vi "CRYChange Curve Library.vi"(4 "Waveform":T1={"Waveform"={"X0"=0.0, "dX"=0.0, "Y"=[]}, "X data"=1, "Y data"=1, "Y axis"=1, "X unit"="s", "Y unit"="V", "Y dB ref"=1.0, "display Y"=TRUE, "display X"=TRUE, "Overload?"=FALSE, "Test Info"="", "Step No."=0, "Name"="", "protected"=FALSE, "Sqc history"=[], "Signal Channel ID"=0, "Plot Settings"={"Color"=0, "Interpolation"=0, "Point Style"=0, "Line Style"=0, "Point Color"=0, "Line Width"=0, "Bar Plot Style"=0, "Fill To"=0}, "AutoProtect"=FALSE} {"Y dB ref" format="%.1f"; "Y axis" items=["Log", "Lin"]; "Y data" items=["dB", "Lin"]; "X data" items=["dB", "Lin"]}, 5 "sOptioin 2":string, 6 "Result":T2={"Name"="Test for Signal [L]", "Margin"=nan, "unit"="", "Verdict"=FALSE, "Limit"="", "Max/Min"="", "protected"=FALSE, "Step No."=0, "Test Info"="", "AutoProtect"=FALSE} {"Margin" format="%.2f"}, 7 "sOptioin 1":string, 8 "Index":i32[](array[numeric]), 9 "Curve":T3={"Name"="", "Curve"=[], "X data"=1, "Y data"=1, "Z data"=1, "X axis"=0, "Y axis"=1, "Z axis"=1, "X unit"="Hz", "Y unit"="", "Z unit"="deg.", "X dB ref"=1.0, "Y dB ref"=1.0, "Z dB ref"=1.0, "single val"=FALSE, "protected"=FALSE, "display X"=TRUE, "display Y"=TRUE, "display Z"=TRUE, "Test Info"="", "Step No."=0, "Plot Settings"={"Color"=0, "Interpolation"=0, "Point Style"=0, "Line Style"=0, "Point Color"=0, "Line Width"=0, "Bar Plot Style"=0, "Fill To"=0}, "AutoProtect"=FALSE} {"Z data" items=["dB", "Lin"]; "X data" items=["dB", "Lin"]; "Y data" items=["dB", "Lin"]; "Z dB ref" format="%.1f"; "Z axis" items=["Log", "Lin"]; "X dB ref" format="%.1f"; "X axis" items=["Log", "Lin"]; "Y axis" items=["Log", "Lin"]; "Y dB ref" format="%.1f"; "Curve"."z" format="%.2f"; "Curve"."y" format="%.2f"; "Curve"."x" format="%.2f"}, 10 "Type In":enum16{"Curves", "Values", "Results", "WFM"}(ring), 11 "sAction":string) -> (2 "Inserted index":i32[](array[numeric]), 3 "Name Out":string[](array[string]))   [LabVIEW 2013]
uses:
  CRYSystem/Typedef Control/CRYData Cluster.ctl
  CRYSystem/Typedef Control/CRYResult Cluster.ctl
  CRYSystem/Typedef Control/CRYWaveform Cluster.ctl
  CRYSystem/Task Sequence/CRYProject Run Control Global.vi
  Global/CRYCurve Library Global.vi
  Global/CRYCurves Array Global.vi
panel:
  # "Save All Data(Curves, Values,Results, Waveforms)"
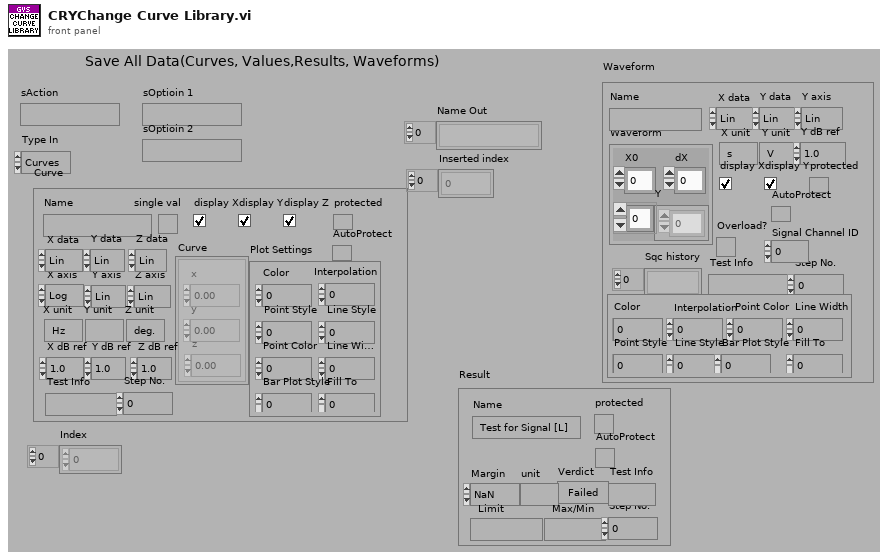
[diagram p1: front panel]
types:
  T1 = typedef "CRYWaveform Cluster.ctl" = cluster{"Waveform":cluster{"X0":dbl, "dX":dbl, "Y":sgl[]}, "X data":u16, "Y data":u16, "Y axis":u16, "X unit":string, "Y unit":string, "Y dB ref":dbl, "display Y":bool, "display X":bool, "Overload?":bool, "Test Info":string, "Step No.":i32, "Name":string, "protected":bool, "Sqc history":string[], "Signal Channel ID":i32, "Plot Settings":cluster{"Color":u32, "Interpolation":u8, "Point Style":u8, "Line Style":u8, "Point Color":u32, "Line Width":u8, "Bar Plot Style":u8, "Fill To":i16}, "AutoProtect":bool}
  T2 = typedef "CRYResult Cluster.ctl" = cluster{"Name":string, "Margin":dbl, "unit":string, "Verdict":bool, "Limit":string, "Max/Min":string, "protected":bool, "Step No.":i32, "Test Info":string, "AutoProtect":bool}
  T3 = typedef "CRYData Cluster.ctl" = cluster{"Name":string, "Curve":cluster{"x":dbl, "y":dbl, "z":dbl}[], "X data":u16, "Y data":u16, "Z data":u16, "X axis":u16, "Y axis":u16, "Z axis":u16, "X unit":string, "Y unit":string, "Z unit":string, "X dB ref":dbl, "Y dB ref":dbl, "Z dB ref":dbl, "single val":bool, "protected":bool, "display X":bool, "display Y":bool, "display Z":bool, "Test Info":string, "Step No.":i32, "Plot Settings":cluster{"Color":u32, "Interpolation":u8, "Point Style":u8, "Line Style":u8, "Point Color":u32, "Line Width":u8, "Bar Plot Style":u8, "Fill To":i16}, "AutoProtect":bool}
  T4 = typedef "CRYWaveform Cluster Array.ctl" = T1[]
  T5 = typedef "CRYResult Cluster Array.ctl" = T2[]
  T6 = typedef "CRYData Cluster Array.ctl" = T3[]
  T7 = cluster{"Color":u32, "Interpolation":u8, "Point Style":u8, "Line Style":u8, "Point Color":u32, "Line Width":u8, "Bar Plot Style":u8, "Fill To":i16}
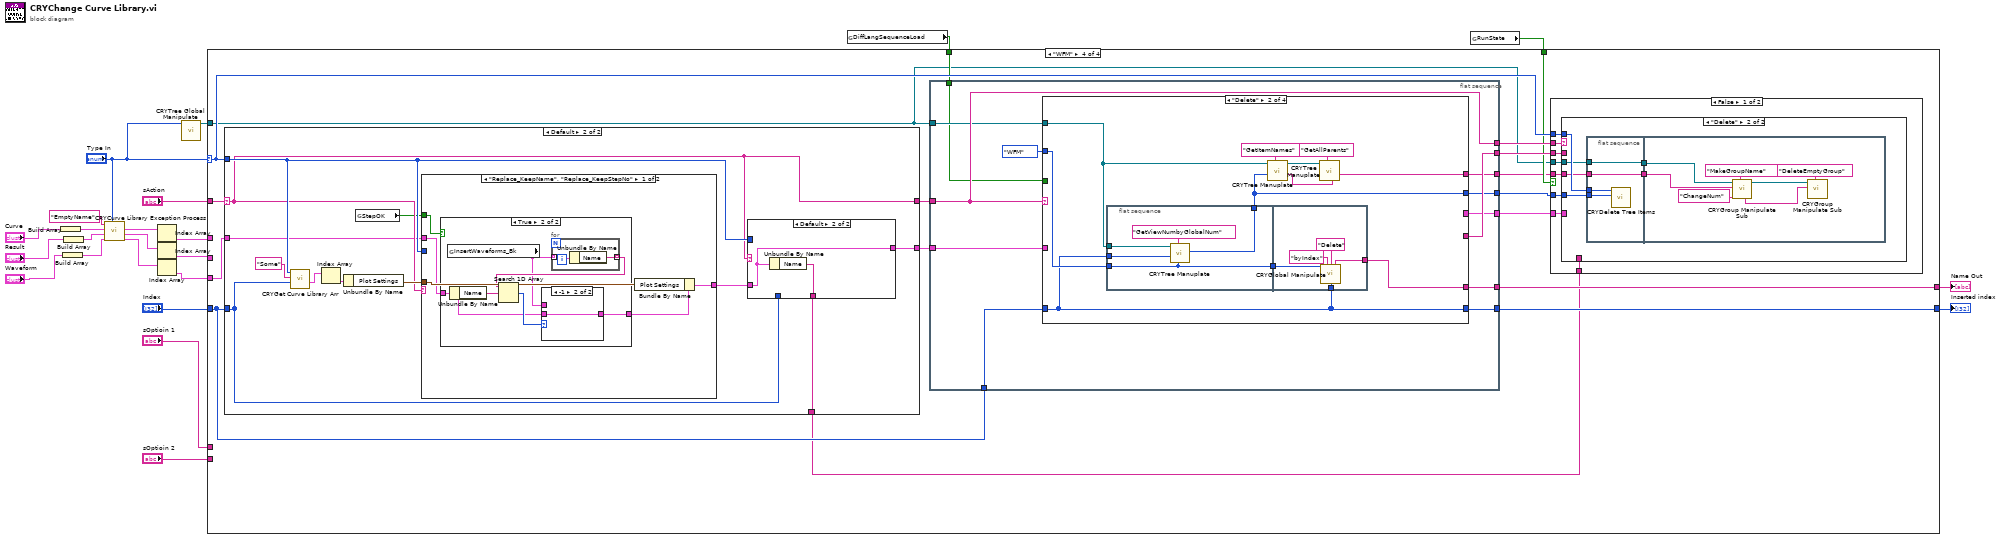
[diagram p0: block diagram]
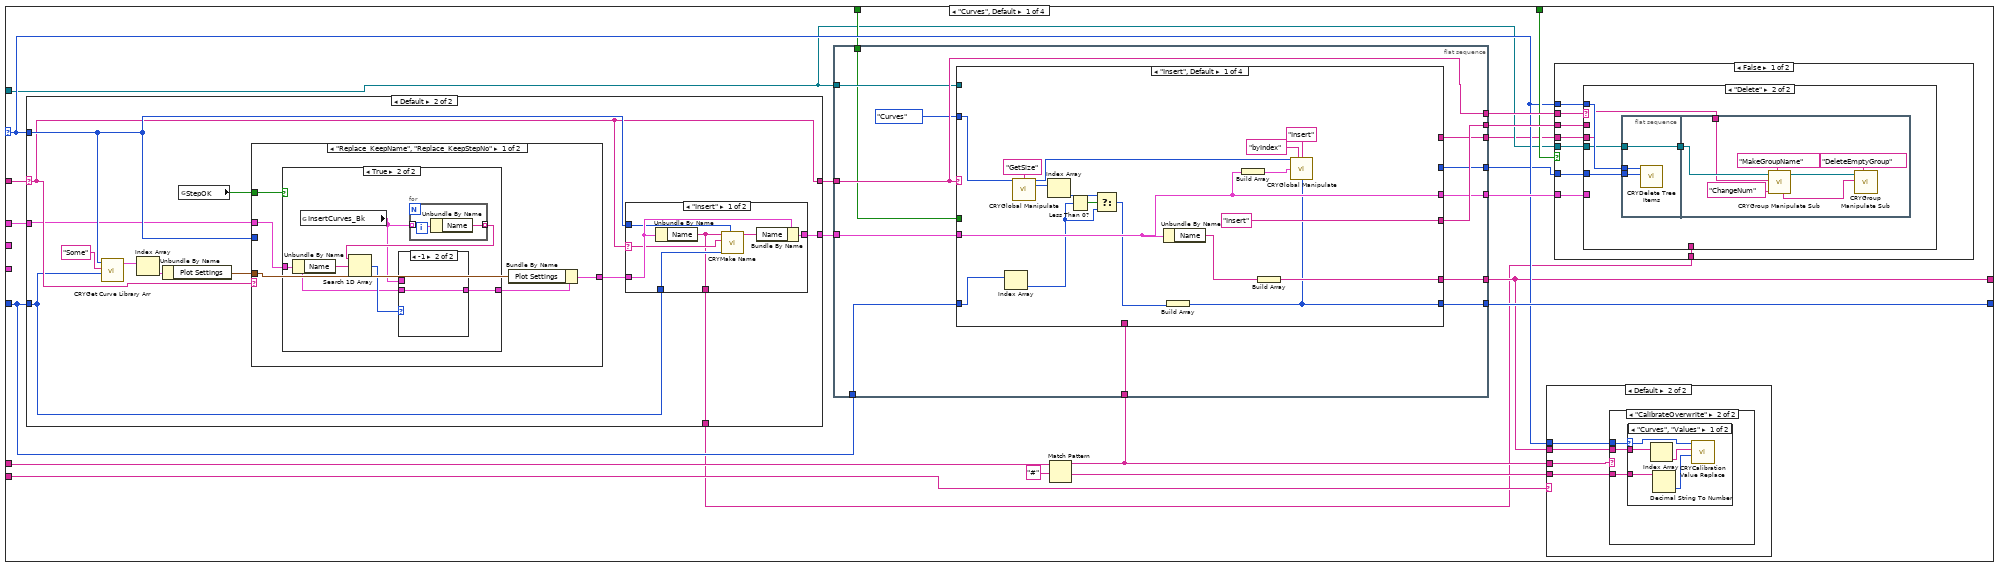
[diagram p2: hidden frame]
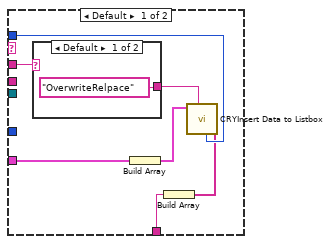
[diagram p6: hidden frame]
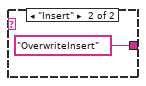
[diagram p7: hidden frame]
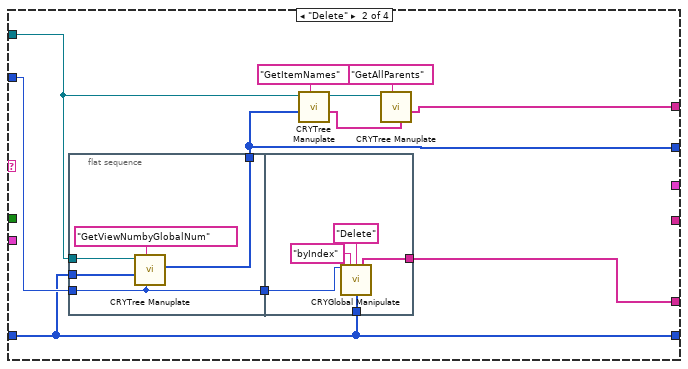
[diagram p9: hidden frame]
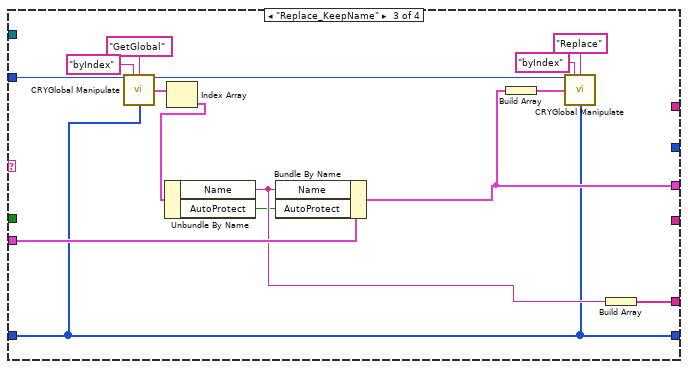
[diagram p10: hidden frame]
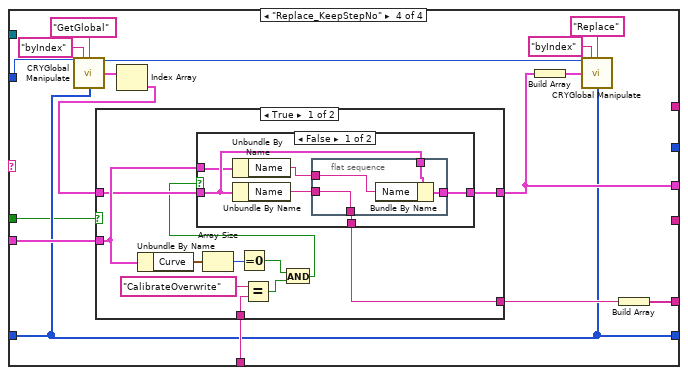
[diagram p11: hidden frame]
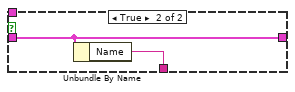
[diagram p12: hidden frame]
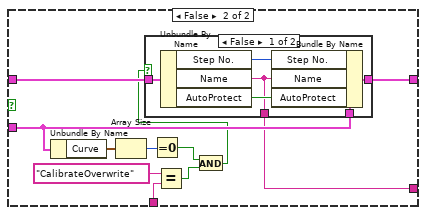
[diagram p13: hidden frame]
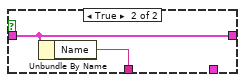
[diagram p14: hidden frame]
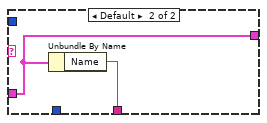
[diagram p16: hidden frame]
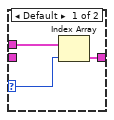
[diagram p18: hidden frame]
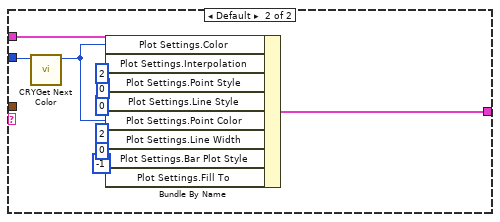
[diagram p19: hidden frame]
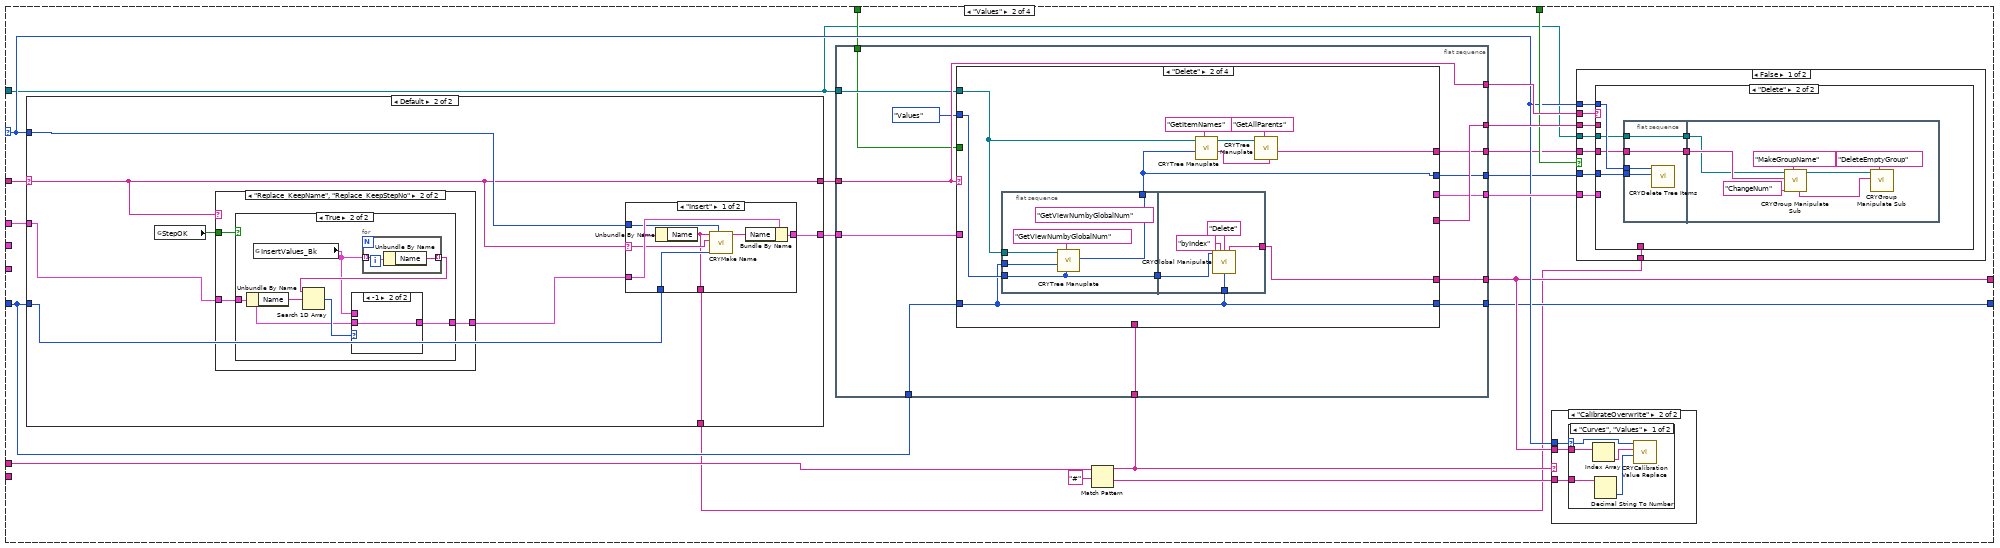
[diagram p20: hidden frame]
diagram:
  n1 = Build Array("Curve") -> (w12:T3[])
  n2 = Build Array("Waveform") -> (w8:T1[])
  n3 = Build Array("Result") -> (w10:T2[])
  n4 = call "CRYCurve Library Exception Process.vi"("Type In"="Type In", "Waveform"=w8, "Result"=w10, "Curve/Value"=w12, "sAction"="EmptyName") -> ("Waveform Out"=w5:T4, "Result Out"=w6:T5, "Curve/Value Out"=w7:T6)  [unwired: 4 in]
  n5 = Index Array(array=w7) -> (element=w4:T3)  [unwired: 1 in]
  n6 = Index Array(array=w6) -> (element=w3:T2)  [unwired: 1 in]
  n7 = Index Array(array=w5) -> (element=w2:T1)  [unwired: 1 in]
  n8 = call "CRYTree Global Manipulate.vi"("Type In"="Type In") -> ("Tree/Curve Tree"=w17:refnum<vi>)  [unwired: 7 in, 3 out]
  n9 = global read "CRYCurve Library Global.vi" "DiffLangSequenceLoad"() -> (w16:bool)
  n10 = global read "CRYProject Run Control Global.vi" "RunState"() -> (w18:bool)
  n11 = case shown="\"WFM\"" "Type In" {
    selector: "Type In" -> [w35 w273 w492 w675]
    tunnel: w4 -> [w45 w284 _ _]
    tunnel: [w39 w269 w497 w679] -> w23
    tunnel: "Index" -> [w43 w282 w501 w683]
    tunnel: "sAction" -> [w42 w281 w500 w682]
    tunnel: [w29 w272 w491 w676] -> w21
    tunnel: "sOptioin 1" -> [w32 w271 _ _]
    tunnel: "sOptioin 2" -> [w34 _ _ _]
    tunnel: w3 -> [_ _ w494 _]
    tunnel: w2 -> [_ _ _ w674]
    tunnel: w18 -> [w36 w276 w493 w673]
    tunnel: w17 -> [w25 w264 w486 w668]
    tunnel: w16 -> [w26 w266 w488 w670]
    frame "Curves", Default {
      n12 = case shown="Default" w42 {
        selector: w42 -> [w214 w219]
        tunnel: w45 -> [_ w218]
        tunnel: [_ w226] -> w44
        tunnel: w43 -> [_ w217]
        tunnel: w35 -> [_ w220]
        tunnel: [w214 w219] -> w41
        tunnel: [_ w216] -> w27
        frame "Delete" {
        }
        frame Default {
          n13 = call "CRYGet Curve Library Arr.vi"("Index"=w217, "sOption"="Some", "Type In"=w220) -> ("Curves/Values"=w224:T6)  [unwired: 6 in, 2 out]
          n14 = Index Array(array=w224) -> (element=w223:T3)  [unwired: 1 in]
          n15 = Unbundle By Name(w223) -> ("Plot Settings"=w222:T7)
          n16 = global read "CRYCurve Library Global.vi" "StepOK"() -> (w215:bool)
          n17 = case shown="\"Replace_KeepName\", \"Replace_KeepStepNo\"" w219 {
            tunnel: w222 -> [w240 _]
            tunnel: w220 -> [_ w263]
            tunnel: [w239 w262] -> w221
            tunnel: w218 -> [w237 w261]
            tunnel: w215 -> [w238 _]
            frame "Replace_KeepName", "Replace_KeepStepNo" {
              n18 = case shown="True" w238 {
                tunnel: w237 -> [w241 w243]
                tunnel: [w241 w242] -> w236
                frame False {
                }
                frame True {
                  n19 = Unbundle By Name(w243) -> ("Name"=w244:string)
                  n20 = global read "CRYCurves Array Global.vi" "InsertCurves_Bk"() -> (w245:T6)
                  n21 = for {
                    tunnel: w245 -> [w253] mode=indexing
                    tunnel: [w252] -> w247 mode=indexing
                    n22 = Unbundle By Name(w253) -> ("Name"=w252:string)
                  }
                  n23 = Search 1D Array(1D array=w247, element=w244) -> (index of element=w246:i32)  [unwired: 1 in]
                  n24 = case shown="-1" w246 {
                    selector: w246 -> [w249 _]
                    tunnel: w245 -> [w250 _]
                    tunnel: [w248 w251] -> w242
                    tunnel: w243 -> [_ w251]
                    frame Default {
                      n25 = Index Array(array=w250, index=w249) -> (element=w248:T3)
                    }
                    frame -1 {
                    }
                  }
                }
              }
              n26 = Bundle By Name(cluster=w236, "Plot Settings"=w240) -> (w239:T3)
            }
            frame Default {
              n27 = call "CRYGet Next Color.vi"("Type"=w263) -> ("Color"=w257:u32)  [unwired: 10 out]
              n28 = Bundle By Name(cluster=w261, "Plot Settings.Color"=w257, "Plot Settings.Interpolation"=u8 2, "Plot Settings.Point Style"=u8 0, "Plot Settings.Line Style"=u8 0, "Plot Settings.Point Color"=w257, "Plot Settings.Line Width"=u8 2, "Plot Settings.Bar Plot Style"=u8 0, "Plot Settings.Fill To"=i16 -1) -> (w262:T3)
            }
          }
          n29 = case shown="\"Insert\"" w219 {
            selector: w219 -> [w229 _]
            tunnel: [w232 w235] -> w226
            tunnel: w221 -> [w231 w235]
            tunnel: w217 -> [w228 _]
            tunnel: w220 -> [w230 _]
            tunnel: [w227 w234] -> w216
            frame "Insert" {
              n30 = Unbundle By Name(w231) -> ("Name"=w227:string)
              n31 = call "CRYMake Name.vi"("Type"=w230, "nData"=w228, "sAction"=w229, "Name In"=w227) -> ("Name Out"=w233:string)  [unwired: 6 in, 1 out]
              n32 = Bundle By Name(cluster=w231, "Name"=w233) -> (w232:T3)
            }
            frame Default {
              n33 = Unbundle By Name(w235) -> ("Name"=w234:string)
            }
          }
        }
      }
      n34 = flat-sequence {
        tunnel: w44 -> [w100]
        tunnel: w43 -> [w94]
        tunnel: w41 -> [w96]
        tunnel: [w96] -> w40
        tunnel: [w101] -> w39
        tunnel: [w99] -> w38
        tunnel: [w98] -> w29
        tunnel: [w102] -> w37
        tunnel: w31 -> [w97]
        tunnel: w25 -> [w93]
        tunnel: [w92] -> w28
        tunnel: w26 -> [w91]
        tunnel: [w90] -> w24
        frame #0 {
          n35 = case shown="\"Insert\", Default" w96 {
            tunnel: w100 -> [w113 _ w155 w171]
            tunnel: w94 -> [w104 w127 w142 w157]
            tunnel: [w109 w127 w142 w157] -> w101
            tunnel: [w113 _ w151 w165] -> w99
            tunnel: [w110 w129 w153 w169] -> w98
            tunnel: ["Insert" ("sOption") _ _ _] -> w102
            tunnel: w97 -> [_ _ _ w168]
            tunnel: enum16{"Curves", "Values", "Results", "WFM"}."Curves" ("Type") -> [w112 w130 w146 w161]
            tunnel: w93 -> [_ w122 _ _]
            tunnel: [_ w121 _ _] -> w92
            tunnel: w91 -> [_ _ _ w156]
            tunnel: [_ w120 _ _] -> w90
            frame "Insert", Default {
              n36 = Index Array(array=w104) -> (element=w106:i32)  [unwired: 1 in]
              n37 = call "CRYGlobal Manipulate.vi"("Type"=w112, "sAction"="GetSize") -> ("Type out"=w111:enum16{"Curves", "Values", "Results", "WFM"}, "nData out"=w116:i32[])  [unwired: 7 in, 5 out]
              n38 = Index Array(array=w116) -> (element=w105:i32)  [unwired: 1 in]
              n39 = Less Than 0?(x=w106) -> (x < 0?=w107:bool)
              n40 = Select(t=w105, s=w107, f=w106) -> (s? t:f=w103:i32)
              n41 = Unbundle By Name(w113) -> ("Name"=w119:string)
              n42 = Build Array(w103) -> (w109:i32[])
              n43 = Build Array(w113) -> (w115:T3[])
              n44 = Build Array(w119) -> (w110:string[])
              n45 = call "CRYGlobal Manipulate.vi"("Type"=w111, "sOption"="byIndex", "sAction"="Insert", "Curves"=w115, "nData"=w109) -> ()  [unwired: 4 in, 7 out]
            }
            frame "Delete" {
              n46 = flat-sequence {
                tunnel: w130 -> [w132]
                tunnel: w122 -> [w134]
                tunnel: w127 -> [w133]
                tunnel: [w132] -> w128
                tunnel: [w131] -> w121
                tunnel: [w138] -> w129
                tunnel: w128 -> [w137]
                tunnel: w127 -> [w136]
                frame #0 {
                  n47 = call "CRYTree Manuplate.vi"("Type"=w132, "sAction"="GetViewNumbyGlobalNum", "nData"=w133, "Tree in"=w134) -> ("nData Out"=w131:i32[])  [unwired: 4 in, 3 out]
                }
                frame #1 {
                  n48 = call "CRYGlobal Manipulate.vi"("Type"=w137, "sOption"="byIndex", "sAction"="Delete", "nData"=w136) -> ("sData Out"=w138:string[])  [unwired: 5 in, 6 out]
                }
              }
              n49 = call "CRYTree Manuplate.vi"("sAction"="GetItemNames", "nData"=w121, "Tree in"=w122) -> ("sData Out"=w123:string[], "Tree Out"=w124:refnum<vi>)  [unwired: 5 in, 2 out]
              n50 = call "CRYTree Manuplate.vi"("sData"=w123, "sAction"="GetAllParents", "Tree in"=w124) -> ("sData Out"=w120:string[])  [unwired: 5 in, 3 out]
            }
            frame "Replace_KeepName" {
              n51 = call "CRYGlobal Manipulate.vi"("Type"=w146, "sOption"="byIndex", "sAction"="GetGlobal", "nData"=w142) -> ("Type out"=w145:enum16{"Curves", "Values", "Results", "WFM"}, "Curves Out"=w148:T3[])  [unwired: 5 in, 5 out]
              n52 = Index Array(array=w148) -> (element=w147:T3)  [unwired: 1 in]
              n53 = Unbundle By Name(w147) -> ("Name"=w154:string, "AutoProtect"=w141:bool)
              n54 = Bundle By Name(cluster=w155, "Name"=w154, "AutoProtect"=w141) -> (w151:T3)
              n55 = Build Array(w151) -> (w150:T3[])
              n56 = call "CRYGlobal Manipulate.vi"("Type"=w145, "sOption"="byIndex", "sAction"="Replace", "Curves"=w150, "nData"=w142) -> ()  [unwired: 4 in, 7 out]
              n57 = Build Array(w154) -> (w153:string[])
            }
            frame "Replace_KeepStepNo" {
              n58 = call "CRYGlobal Manipulate.vi"("Type"=w161, "sOption"="byIndex", "sAction"="GetGlobal", "nData"=w157) -> ("Type out"=w160:enum16{"Curves", "Values", "Results", "WFM"}, "Curves Out"=w163:T3[])  [unwired: 5 in, 5 out]
              n59 = Index Array(array=w163) -> (element=w162:T3)  [unwired: 1 in]
              n60 = case shown="True" w156 {
                tunnel: w171 -> [w182 w205]
                tunnel: [w181 w204] -> w170
                tunnel: w168 -> [w180 w203]
                tunnel: [w179 w202] -> w165
                tunnel: w162 -> [w178 w201]
                frame True {
                  n61 = Unbundle By Name(w182) -> ("Curve"=w177:cluster{"x":dbl, "y":dbl, "z":dbl}[])
                  n62 = Array Size(array=w177) -> (size(s)=w176:i32)
                  n63 = Equal To 0?(x=w176) -> (x = 0?=w173:bool)
                  n64 = Equal?(x="CalibrateOverwrite", y=w180) -> (x = y?=w174:bool)
                  n65 = And(x=w173, y=w174) -> (x .and. y?=w172:bool)
                  n66 = case shown="False" w172 {
                    tunnel: w178 -> [w187 w194]
                    tunnel: [w184 w193] -> w181
                    tunnel: [w188 w194] -> w179
                    tunnel: w182 -> [w186 _]
                    frame False {
                      n67 = Unbundle By Name(w186) -> ("Name"=w185:string)
                      n68 = Unbundle By Name(w187) -> ("Name"=w183:string)
                      n69 = flat-sequence {
                        tunnel: [w192] -> w188
                        tunnel: w187 -> [w191]
                        tunnel: w185 -> [w190]
                        tunnel: [w189] -> w184
                        tunnel: w183 -> [w189]
                        frame #0 {
                          n70 = Bundle By Name(cluster=w191, "Name"=w190) -> (w192:T3)
                        }
                      }
                    }
                    frame True {
                      n71 = Unbundle By Name(w194) -> ("Name"=w193:string)
                    }
                  }
                }
                frame False {
                  n72 = Unbundle By Name(w205) -> ("Curve"=w200:cluster{"x":dbl, "y":dbl, "z":dbl}[])
                  n73 = Array Size(array=w200) -> (size(s)=w199:i32)
                  n74 = Equal To 0?(x=w199) -> (x = 0?=w196:bool)
                  n75 = Equal?(x="CalibrateOverwrite", y=w203) -> (x = y?=w197:bool)
                  n76 = And(x=w196, y=w197) -> (x .and. y?=w195:bool)
                  n77 = case shown="False" w195 {
                    tunnel: w201 -> [w210 w213]
                    tunnel: [w209 w212] -> w204
                    tunnel: [w208 w213] -> w202
                    tunnel: w205 -> [w206 _]
                    frame False {
                      n78 = Unbundle By Name(w210) -> ("Step No."=w207:i32, "Name"=w209:string, "AutoProtect"=w211:bool)
                      n79 = Bundle By Name(cluster=w206, "Step No."=w207, "Name"=w209, "AutoProtect"=w211) -> (w208:T3)
                    }
                    frame True {
                      n80 = Unbundle By Name(w213) -> ("Name"=w212:string)
                    }
                  }
                }
              }
              n81 = Build Array(w165) -> (w166:T3[])
              n82 = call "CRYGlobal Manipulate.vi"("Type"=w160, "sOption"="byIndex", "sAction"="Replace", "Curves"=w166, "nData"=w157) -> ()  [unwired: 4 in, 7 out]
              n83 = Build Array(w170) -> (w169:string[])
            }
          }
        }
      }
      n84 = Match Pattern(string=w32, regular expression="#" ("string")) -> (before substring=w31:string, after substring=w30:string)  [unwired: 1 in, 2 out]
      n85 = case shown="Default" w34 {
        tunnel: w35 -> [_ w49]
        tunnel: w31 -> [_ w46]
        tunnel: w29 -> [_ w48]
        tunnel: w30 -> [_ w47]
        frame "CalibrateOverwrite_NoCalSignal" {
        }
        frame Default {
          n86 = case shown="\"CalibrateOverwrite\"" w46 {
            tunnel: w48 -> [_ w52]
            tunnel: w49 -> [_ w51]
            tunnel: w47 -> [_ w50]
            frame Default {
            }
            frame "CalibrateOverwrite" {
              n87 = case shown="\"Curves\", \"Values\"" w51 {
                selector: w51 -> [w55 _]
                tunnel: w52 -> [w54 _]
                tunnel: w50 -> [w57 _]
                frame "Curves", "Values" {
                  n88 = Index Array(array=w54) -> (element=w53:string)  [unwired: 1 in]
                  n89 = Decimal String To Number(string=w57) -> (number=w56:i32)  [unwired: 2 in, 1 out]
                  n90 = call "CRYCalibration Value Replace.vi"("Step No."=w56, "Corr/EQ/Sens Name"=w53, "Type"=w55) -> ()  [unwired: 9 in]
                }
                frame Default {
                }
              }
            }
          }
        }
      }
      n91 = case shown="False" w36 {
        tunnel: w40 -> [w65 _]
        tunnel: w28 -> [w64 _]
        tunnel: w38 -> [w63 _]
        tunnel: w37 -> [w62 _]
        tunnel: w35 -> [w61 _]
        tunnel: w27 -> [w60 _]
        tunnel: w25 -> [w59 _]
        tunnel: w24 -> [w58 _]
        frame False {
          n92 = case shown="\"Delete\"" w65 {
            tunnel: w61 -> [w68 w79]
            tunnel: w64 -> [_ w78]
            tunnel: w63 -> [w72 _]
            tunnel: w62 -> [w69 _]
            tunnel: w60 -> [w67 _]
            tunnel: w59 -> [_ w77]
            tunnel: w58 -> [_ w75]
            frame Default {
              n93 = case shown="Default" w69 {
                tunnel: ["OverwriteRelpace" ("sOption") "OverwriteInsert" ("sOption")] -> w70
                frame Default {
                }
                frame "Insert" {
                }
              }
              n94 = Build Array(w72) -> (w71:T3[])
              n95 = Build Array(w67) -> (w66:string[])
              n96 = call "CRYInsert Data to Listbox.vi"("OrgNames"=w66, "Type"=w68, "sOption"=w70, "Curves"=w71) -> ()  [unwired: 7 in, 1 out]
            }
            frame "Delete" {
              n97 = flat-sequence {
                tunnel: w79 -> [w82]
                tunnel: w78 -> [w81]
                tunnel: w77 -> [w80]
                tunnel: [w80] -> w76
                tunnel: w76 -> [w84]
                tunnel: w75 -> [w83]
                frame #0 {
                  n98 = call "CRYDelete Tree Items.vi"("Array"=w81, "Type"=w82) -> ()  [unwired: 2 in, 8 out]
                }
                frame #1 {
                  n99 = call "CRYGroup Manipulate Sub.vi"("sAction"="MakeGroupName", "sOption"="ChangeNum", "sData"=w83, "Tree in"=w84) -> ("Tree Out"=w86:refnum<vi>, "sData Out"=w85:string[])  [unwired: 3 in, 3 out]
                  n100 = call "CRYGroup Manipulate Sub.vi"("sAction"="DeleteEmptyGroup", "sData"=w85, "Tree in"=w86) -> ()  [unwired: 4 in, 5 out]
                }
              }
            }
          }
        }
        frame True {
        }
      }
    }
    frame "Values" {
      n101 = case shown="Default" w281 {
        selector: w281 -> [w451 w454]
        tunnel: w284 -> [_ w453]
        tunnel: [_ w459] -> w283
        tunnel: w282 -> [_ w458]
        tunnel: w273 -> [_ w457]
        tunnel: [w451 w454] -> w280
        tunnel: [_ w456] -> w267
        frame "Delete" {
        }
        frame Default {
          n102 = global read "CRYCurve Library Global.vi" "StepOK"() -> (w455:bool)
          n103 = case shown="\"Replace_KeepName\", \"Replace_KeepStepNo\"" w454 {
            tunnel: w455 -> [_ w463]
            tunnel: w453 -> [w460 w462]
            tunnel: [w460 w461] -> w452
            frame Default {
            }
            frame "Replace_KeepName", "Replace_KeepStepNo" {
              n104 = case shown="True" w463 {
                tunnel: w462 -> [w464 w466]
                tunnel: [w464 w465] -> w461
                frame False {
                }
                frame True {
                  n105 = Unbundle By Name(w466) -> ("Name"=w467:string)
                  n106 = global read "CRYCurves Array Global.vi" "InsertValues_Bk"() -> (w468:T6)
                  n107 = for {
                    tunnel: w468 -> [w476] mode=indexing
                    tunnel: [w475] -> w470 mode=indexing
                    n108 = Unbundle By Name(w476) -> ("Name"=w475:string)
                  }
                  n109 = Search 1D Array(1D array=w470, element=w467) -> (index of element=w469:i32)  [unwired: 1 in]
                  n110 = case shown="-1" w469 {
                    selector: w469 -> [w472 _]
                    tunnel: w468 -> [w473 _]
                    tunnel: [w471 w474] -> w465
                    tunnel: w466 -> [_ w474]
                    frame Default {
                      n111 = Index Array(array=w473, index=w472) -> (element=w471:T3)
                    }
                    frame -1 {
                    }
                  }
                }
              }
            }
          }
          n112 = case shown="\"Insert\"" w454 {
            selector: w454 -> [w479 _]
            tunnel: [w482 w485] -> w459
            tunnel: w452 -> [w481 w485]
            tunnel: w458 -> [w478 _]
            tunnel: w457 -> [w480 _]
            tunnel: [w477 w484] -> w456
            frame "Insert" {
              n113 = Unbundle By Name(w481) -> ("Name"=w477:string)
              n114 = call "CRYMake Name.vi"("Type"=w480, "nData"=w478, "sAction"=w479, "Name In"=w477) -> ("Name Out"=w483:string)  [unwired: 6 in, 1 out]
              n115 = Bundle By Name(cluster=w481, "Name"=w483) -> (w482:T3)
            }
            frame Default {
              n116 = Unbundle By Name(w485) -> ("Name"=w484:string)
            }
          }
        }
      }
      n117 = flat-sequence {
        tunnel: w283 -> [w337]
        tunnel: w282 -> [w331]
        tunnel: w280 -> [w333]
        tunnel: [w333] -> w279
        tunnel: [w338] -> w269
        tunnel: [w336] -> w278
        tunnel: [w335] -> w272
        tunnel: [w339] -> w277
        tunnel: w270 -> [w334]
        tunnel: w264 -> [w330]
        tunnel: [w329] -> w268
        tunnel: w266 -> [w328]
        tunnel: [w327] -> w265
        frame #0 {
          n118 = case shown="\"Delete\"" w333 {
            tunnel: w337 -> [w348 _ w392 w408]
            tunnel: w331 -> [w352 w364 w380 w395]
            tunnel: [w341 w364 w380 w395] -> w338
            tunnel: [w348 _ w386 w400] -> w336
            tunnel: [w350 w366 w390 w406] -> w335
            tunnel: ["Insert" ("sOption") _ _ _] -> w339
            tunnel: w334 -> [_ _ _ w405]
            tunnel: enum16{"Curves", "Values", "Results", "WFM"}."Values" ("Type") -> [w342 w365 w382 w397]
            tunnel: w330 -> [_ w358 _ _]
            tunnel: [_ w359 _ _] -> w329
            tunnel: w328 -> [_ _ _ w393]
            tunnel: [_ w357 _ _] -> w327
            frame "Insert", Default {
              n119 = Index Array(array=w352) -> (element=w351:i32)  [unwired: 1 in]
              n120 = call "CRYGlobal Manipulate.vi"("Type"=w342, "sAction"="GetSize") -> ("Type out"=w344:enum16{"Curves", "Values", "Results", "WFM"}, "nData out"=w347:i32[])  [unwired: 7 in, 5 out]
              n121 = Index Array(array=w347) -> (element=w345:i32)  [unwired: 1 in]
              n122 = Less Than 0?(x=w351) -> (x < 0?=w356:bool)
              n123 = Select(t=w345, s=w356, f=w351) -> (s? t:f=w353:i32)
              n124 = Build Array(w353) -> (w341:i32[])
              n125 = Unbundle By Name(w348) -> ("Name"=w355:string)
              n126 = Build Array(w348) -> (w343:T3[])
              n127 = call "CRYGlobal Manipulate.vi"("Type"=w344, "sOption"="byIndex", "sAction"="Insert", "Values"=w343, "nData"=w341) -> ()  [unwired: 4 in, 7 out]
              n128 = Build Array(w355) -> (w350:string[])
            }
            frame "Delete" {
              (unwired) "GetViewNumbyGlobalNum" ("sAction")
              n129 = flat-sequence {
                tunnel: w365 -> [w369]
                tunnel: w358 -> [w371]
                tunnel: w364 -> [w370]
                tunnel: [w369] -> w367
                tunnel: [w368] -> w359
                tunnel: [w375] -> w366
                tunnel: w367 -> [w374]
                tunnel: w364 -> [w373]
                frame #0 {
                  n130 = call "CRYTree Manuplate.vi"("Type"=w369, "sAction"="GetViewNumbyGlobalNum", "nData"=w370, "Tree in"=w371) -> ("nData Out"=w368:i32[])  [unwired: 4 in, 3 out]
                }
                frame #1 {
                  n131 = call "CRYGlobal Manipulate.vi"("Type"=w374, "sOption"="byIndex", "sAction"="Delete", "nData"=w373) -> ("sData Out"=w375:string[])  [unwired: 5 in, 6 out]
                }
              }
              n132 = call "CRYTree Manuplate.vi"("sAction"="GetItemNames", "nData"=w359, "Tree in"=w358) -> ("sData Out"=w360:string[], "Tree Out"=w361:refnum<vi>)  [unwired: 5 in, 2 out]
              n133 = call "CRYTree Manuplate.vi"("sData"=w360, "sAction"="GetAllParents", "Tree in"=w361) -> ("sData Out"=w357:string[])  [unwired: 5 in, 3 out]
            }
            frame "Replace_KeepName" {
              n134 = call "CRYGlobal Manipulate.vi"("Type"=w382, "sOption"="byIndex", "sAction"="GetGlobal", "nData"=w380) -> ("Type out"=w385:enum16{"Curves", "Values", "Results", "WFM"}, "Values Out"=w383:T3[])  [unwired: 5 in, 5 out]
              n135 = Index Array(array=w383) -> (element=w388:T3)  [unwired: 1 in]
              n136 = Unbundle By Name(w388) -> ("Name"=w391:string, "AutoProtect"=w378:bool)
              n137 = Bundle By Name(cluster=w392, "Name"=w391, "AutoProtect"=w378) -> (w386:T3)
              n138 = Build Array(w386) -> (w384:T3[])
              n139 = Build Array(w391) -> (w390:string[])
              n140 = call "CRYGlobal Manipulate.vi"("Type"=w385, "sOption"="byIndex", "sAction"="Replace", "Values"=w384, "nData"=w380) -> ()  [unwired: 4 in, 7 out]
            }
            frame "Replace_KeepStepNo" {
              n141 = call "CRYGlobal Manipulate.vi"("Type"=w397, "sOption"="byIndex", "sAction"="GetGlobal", "nData"=w395) -> ("Type out"=w402:enum16{"Curves", "Values", "Results", "WFM"}, "Values Out"=w399:T3[])  [unwired: 5 in, 5 out]
              n142 = Index Array(array=w399) -> (element=w401:T3)  [unwired: 1 in]
              n143 = case shown="True" w393 {
                tunnel: w408 -> [w419 w442]
                tunnel: [w418 w441] -> w407
                tunnel: w405 -> [w417 w440]
                tunnel: w401 -> [w416 w439]
                tunnel: [w415 w438] -> w400
                frame True {
                  n144 = Unbundle By Name(w419) -> ("Curve"=w414:cluster{"x":dbl, "y":dbl, "z":dbl}[])
                  n145 = Array Size(array=w414) -> (size(s)=w413:i32)
                  n146 = Equal To 0?(x=w413) -> (x = 0?=w410:bool)
                  n147 = Equal?(x="CalibrateOverwrite", y=w417) -> (x = y?=w411:bool)
                  n148 = And(x=w410, y=w411) -> (x .and. y?=w409:bool)
                  n149 = case shown="False" w409 {
                    tunnel: w416 -> [w423 w431]
                    tunnel: [w421 w430] -> w418
                    tunnel: [w425 w431] -> w415
                    tunnel: w419 -> [w424 _]
                    frame False {
                      n150 = Unbundle By Name(w424) -> ("Name"=w422:string)
                      n151 = Unbundle By Name(w423) -> ("Name"=w420:string)
                      n152 = flat-sequence {
                        tunnel: [w429] -> w425
                        tunnel: w423 -> [w428]
                        tunnel: w422 -> [w427]
                        tunnel: [w426] -> w421
                        tunnel: w420 -> [w426]
                        frame #0 {
                          n153 = Bundle By Name(cluster=w428, "Name"=w427) -> (w429:T3)
                        }
                      }
                    }
                    frame True {
                      n154 = Unbundle By Name(w431) -> ("Name"=w430:string)
                    }
                  }
                }
                frame False {
                  n155 = Unbundle By Name(w442) -> ("Curve"=w437:cluster{"x":dbl, "y":dbl, "z":dbl}[])
                  n156 = Array Size(array=w437) -> (size(s)=w436:i32)
                  n157 = Equal To 0?(x=w436) -> (x = 0?=w433:bool)
                  n158 = Equal?(x="CalibrateOverwrite", y=w440) -> (x = y?=w434:bool)
                  n159 = And(x=w433, y=w434) -> (x .and. y?=w432:bool)
                  n160 = case shown="False" w432 {
                    tunnel: w439 -> [w447 w450]
                    tunnel: [w446 w449] -> w441
                    tunnel: [w445 w450] -> w438
                    tunnel: w442 -> [w443 _]
                    frame False {
                      n161 = Unbundle By Name(w447) -> ("Step No."=w444:i32, "Name"=w446:string, "AutoProtect"=w448:bool)
                      n162 = Bundle By Name(cluster=w443, "Step No."=w444, "Name"=w446, "AutoProtect"=w448) -> (w445:T3)
                    }
                    frame True {
                      n163 = Unbundle By Name(w450) -> ("Name"=w449:string)
                    }
                  }
                }
              }
              n164 = Build Array(w400) -> (w398:T3[])
              n165 = call "CRYGlobal Manipulate.vi"("Type"=w402, "sOption"="byIndex", "sAction"="Replace", "Values"=w398, "nData"=w395) -> ()  [unwired: 4 in, 7 out]
              n166 = Build Array(w407) -> (w406:string[])
            }
          }
        }
      }
      n167 = Match Pattern(string=w271, regular expression="#" ("string")) -> (before substring=w270:string, after substring=w274:string)  [unwired: 1 in, 2 out]
      n168 = case shown="\"CalibrateOverwrite\"" w270 {
        tunnel: w272 -> [_ w287]
        tunnel: w273 -> [_ w286]
        tunnel: w274 -> [_ w285]
        frame Default {
        }
        frame "CalibrateOverwrite" {
          n169 = case shown="\"Curves\", \"Values\"" w286 {
            selector: w286 -> [w290 _]
            tunnel: w287 -> [w289 _]
            tunnel: w285 -> [w292 _]
            frame "Curves", "Values" {
              n170 = Index Array(array=w289) -> (element=w288:string)  [unwired: 1 in]
              n171 = Decimal String To Number(string=w292) -> (number=w291:i32)  [unwired: 2 in, 1 out]
              n172 = call "CRYCalibration Value Replace.vi"("Step No."=w291, "Corr/EQ/Sens Name"=w288, "Type"=w290) -> ()  [unwired: 9 in]
            }
            frame Default {
            }
          }
        }
      }
      n173 = case shown="False" w276 {
        tunnel: w279 -> [w300 _]
        tunnel: w268 -> [w299 _]
        tunnel: w278 -> [w298 _]
        tunnel: w277 -> [w297 _]
        tunnel: w273 -> [w296 _]
        tunnel: w267 -> [w295 _]
        tunnel: w265 -> [w294 _]
        tunnel: w264 -> [w293 _]
        frame False {
          n174 = case shown="\"Delete\"" w300 {
            tunnel: w296 -> [w304 w315]
            tunnel: w299 -> [_ w314]
            tunnel: w298 -> [w307 _]
            tunnel: w297 -> [w305 _]
            tunnel: w295 -> [w302 _]
            tunnel: w294 -> [_ w312]
            tunnel: w293 -> [_ w310]
            frame Default {
              n175 = case shown="Default" w305 {
                tunnel: ["OverwriteRelpace" ("sOption") "OverwriteInsert" ("sOption")] -> w306
                frame Default {
                }
                frame "Insert" {
                }
              }
              n176 = Build Array(w307) -> (w303:T3[])
              n177 = Build Array(w302) -> (w301:string[])
              n178 = call "CRYInsert Data to Listbox.vi"("OrgNames"=w301, "Type"=w304, "sOption"=w306, "Values"=w303) -> ()  [unwired: 7 in, 1 out]
            }
            frame "Delete" {
              n179 = flat-sequence {
                tunnel: w315 -> [w319]
                tunnel: w314 -> [w318]
                tunnel: [w317] -> w313
                tunnel: w312 -> [w317]
                tunnel: [w316] -> w311
                tunnel: w310 -> [w316]
                tunnel: w313 -> [w321]
                tunnel: w311 -> [w320]
                frame #0 {
                  n180 = call "CRYDelete Tree Items.vi"("Array"=w318, "Type"=w319) -> ()  [unwired: 2 in, 8 out]
                }
                frame #1 {
                  n181 = call "CRYGroup Manipulate Sub.vi"("sAction"="MakeGroupName", "sOption"="ChangeNum", "sData"=w321, "Tree in"=w320) -> ("Tree Out"=w325:refnum<vi>, "sData Out"=w326:string[])  [unwired: 3 in, 3 out]
                  n182 = call "CRYGroup Manipulate Sub.vi"("sAction"="DeleteEmptyGroup", "sData"=w326, "Tree in"=w325) -> ()  [unwired: 4 in, 5 out]
                }
              }
            }
          }
        }
        frame True {
        }
      }
    }
    frame "Results" {
      n183 = case shown="Default" w500 {
        selector: w500 -> [w633 w636]
        tunnel: w494 -> [_ w635]
        tunnel: [_ w641] -> w502
        tunnel: w501 -> [_ w640]
        tunnel: w492 -> [_ w639]
        tunnel: [w633 w636] -> w499
        tunnel: [_ w638] -> w489
        frame "Delete" {
        }
        frame Default {
          n184 = global read "CRYCurve Library Global.vi" "StepOK"() -> (w637:bool)
          n185 = case shown="Default" w636 {
            tunnel: w637 -> [_ w645]
            tunnel: w635 -> [w642 w644]
            tunnel: [w642 w643] -> w634
            frame Default {
            }
            frame "Replace_KeepName", "Replace_KeepStepNo" {
              n186 = case shown="True" w645 {
                tunnel: w644 -> [w646 w648]
                tunnel: [w646 w647] -> w643
                frame False {
                }
                frame True {
                  n187 = Unbundle By Name(w648) -> ("Name"=w649:string)
                  n188 = global read "CRYCurves Array Global.vi" "InsertResults_Bk"() -> (w650:T5)
                  n189 = for {
                    tunnel: w650 -> [w658] mode=indexing
                    tunnel: [w657] -> w652 mode=indexing
                    n190 = Unbundle By Name(w658) -> ("Name"=w657:string)
                  }
                  n191 = Search 1D Array(1D array=w652, element=w649) -> (index of element=w651:i32)  [unwired: 1 in]
                  n192 = case shown="-1" w651 {
                    selector: w651 -> [w654 _]
                    tunnel: w650 -> [w655 _]
                    tunnel: [w653 w656] -> w647
                    tunnel: w648 -> [_ w656]
                    frame Default {
                      n193 = Index Array(array=w655, index=w654) -> (element=w653:T2)
                    }
                    frame -1 {
                    }
                  }
                }
              }
            }
          }
          n194 = case shown="Default" w636 {
            selector: w636 -> [w661 _]
            tunnel: [w664 w667] -> w641
            tunnel: w634 -> [w663 w667]
            tunnel: w640 -> [w660 _]
            tunnel: w639 -> [w662 _]
            tunnel: [w659 w666] -> w638
            frame "Insert" {
              n195 = Unbundle By Name(w663) -> ("Name"=w659:string)
              n196 = call "CRYMake Name.vi"("Type"=w662, "nData"=w660, "sAction"=w661, "Name In"=w659) -> ("Name Out"=w665:string)  [unwired: 6 in, 1 out]
              n197 = Bundle By Name(cluster=w663, "Name"=w665) -> (w664:T2)
            }
            frame Default {
              n198 = Unbundle By Name(w667) -> ("Name"=w666:string)
            }
          }
        }
      }
      n199 = flat-sequence {
        tunnel: w502 -> [w546]
        tunnel: w501 -> [w541]
        tunnel: w499 -> [w543]
        tunnel: [w543] -> w498
        tunnel: [w547] -> w497
        tunnel: [w545] -> w496
        tunnel: [w544] -> w491
        tunnel: [w548] -> w495
        tunnel: w486 -> [w540]
        tunnel: [w539] -> w490
        tunnel: w488 -> [w538]
        tunnel: [w537] -> w487
        frame #0 {
          n200 = case shown="\"Insert\", Default" w543 {
            tunnel: w546 -> [w554 _ w601 w616]
            tunnel: w541 -> [w561 w573 w589 w604]
            tunnel: [w550 w573 w589 w604] -> w547
            tunnel: [w554 _ w595 w608] -> w545
            tunnel: [w559 w574 w590 w614] -> w544
            tunnel: ["Insert" ("sOption") _ _ _] -> w548
            tunnel: enum16{"Curves", "Values", "Results", "WFM"}."Results" ("Type") -> [w551 w575 w592 w606]
            tunnel: w540 -> [_ w568 _ _]
            tunnel: [_ w567 _ _] -> w539
            tunnel: w538 -> [_ _ _ w602]
            tunnel: [_ w566 _ _] -> w537
            frame "Insert", Default {
              n201 = call "CRYGlobal Manipulate.vi"("Type"=w551, "sAction"="GetSize") -> ("Type out"=w552:enum16{"Curves", "Values", "Results", "WFM"}, "nData out"=w558:i32[])  [unwired: 7 in, 5 out]
              n202 = Index Array(array=w561) -> (element=w560:i32)  [unwired: 1 in]
              n203 = Index Array(array=w558) -> (element=w556:i32)  [unwired: 1 in]
              n204 = Less Than 0?(x=w560) -> (x < 0?=w565:bool)
              n205 = Select(t=w556, s=w565, f=w560) -> (s? t:f=w562:i32)
              n206 = Build Array(w562) -> (w550:i32[])
              n207 = Unbundle By Name(w554) -> ("Name"=w564:string)
              n208 = Build Array(w554) -> (w553:T2[])
              n209 = Build Array(w564) -> (w559:string[])
              n210 = call "CRYGlobal Manipulate.vi"("Type"=w552, "sOption"="byIndex", "sAction"="Insert", "Results"=w553, "nData"=w550) -> ()  [unwired: 4 in, 7 out]
            }
            frame "Delete" {
              n211 = flat-sequence {
                tunnel: w575 -> [w578]
                tunnel: w568 -> [w580]
                tunnel: w573 -> [w579]
                tunnel: [w578] -> w576
                tunnel: [w577] -> w567
                tunnel: [w584] -> w574
                tunnel: w576 -> [w583]
                tunnel: w573 -> [w582]
                frame #0 {
                  n212 = call "CRYTree Manuplate.vi"("Type"=w578, "sAction"="GetViewNumbyGlobalNum", "nData"=w579, "Tree in"=w580) -> ("nData Out"=w577:i32[])  [unwired: 4 in, 3 out]
                }
                frame #1 {
                  n213 = call "CRYGlobal Manipulate.vi"("Type"=w583, "sOption"="byIndex", "sAction"="Delete", "nData"=w582) -> ("sData Out"=w584:string[])  [unwired: 5 in, 6 out]
                }
              }
              n214 = call "CRYTree Manuplate.vi"("sAction"="GetItemNames", "nData"=w567, "Tree in"=w568) -> ("sData Out"=w569:string[], "Tree Out"=w570:refnum<vi>)  [unwired: 5 in, 2 out]
              n215 = call "CRYTree Manuplate.vi"("sData"=w569, "sAction"="GetAllParents", "Tree in"=w570) -> ("sData Out"=w566:string[])  [unwired: 5 in, 3 out]
            }
            frame "Replace_KeepName" {
              n216 = call "CRYGlobal Manipulate.vi"("Type"=w592, "sOption"="byIndex", "sAction"="GetGlobal", "nData"=w589) -> ("Type out"=w596:enum16{"Curves", "Values", "Results", "WFM"}, "Results Out"=w598:T2[])  [unwired: 5 in, 5 out]
              n217 = Index Array(array=w598) -> (element=w594:T2)  [unwired: 1 in]
              n218 = Unbundle By Name(w594) -> ("Name"=w600:string, "AutoProtect"=w587:bool)
              n219 = Bundle By Name(cluster=w601, "Name"=w600, "AutoProtect"=w587) -> (w595:T2)
              n220 = Build Array(w595) -> (w593:T2[])
              n221 = call "CRYGlobal Manipulate.vi"("Type"=w596, "sOption"="byIndex", "sAction"="Replace", "Results"=w593, "nData"=w589) -> ()  [unwired: 4 in, 7 out]
              n222 = Build Array(w600) -> (w590:string[])
            }
            frame "Replace_KeepStepNo" {
              n223 = call "CRYGlobal Manipulate.vi"("Type"=w606, "sOption"="byIndex", "sAction"="GetGlobal", "nData"=w604) -> ("Type out"=w611:enum16{"Curves", "Values", "Results", "WFM"}, "Results Out"=w609:T2[])  [unwired: 5 in, 5 out]
              n224 = Index Array(array=w609) -> (element=w610:T2)  [unwired: 1 in]
              n225 = case shown="True" w602 {
                tunnel: w616 -> [w621 w632]
                tunnel: [w619 w631] -> w615
                tunnel: w610 -> [w617 w630]
                tunnel: [w622 w629] -> w608
                frame True {
                  n226 = Unbundle By Name(w621) -> ("Name"=w620:string)
                  n227 = Unbundle By Name(w617) -> ("Name"=w618:string)
                  n228 = flat-sequence {
                    tunnel: [w626] -> w622
                    tunnel: w620 -> [w625]
                    tunnel: [w624] -> w619
                    tunnel: w618 -> [w624]
                    tunnel: w617 -> [w623]
                    frame #0 {
                      n229 = Bundle By Name(cluster=w623, "Name"=w625) -> (w626:T2)
                    }
                  }
                }
                frame False {
                  n230 = Unbundle By Name(w630) -> ("Step No."=w627:i32, "Name"=w631:string, "AutoProtect"=w628:bool)
                  n231 = Bundle By Name(cluster=w632, "Step No."=w627, "Name"=w631, "AutoProtect"=w628) -> (w629:T2)
                }
              }
              n232 = Build Array(w608) -> (w607:T2[])
              n233 = call "CRYGlobal Manipulate.vi"("Type"=w611, "sOption"="byIndex", "sAction"="Replace", "Results"=w607, "nData"=w604) -> ()  [unwired: 4 in, 7 out]
              n234 = Build Array(w615) -> (w614:string[])
            }
          }
        }
      }
      n235 = case shown="False" w493 {
        tunnel: w498 -> [w510 _]
        tunnel: w490 -> [w509 _]
        tunnel: w496 -> [w508 _]
        tunnel: w495 -> [w507 _]
        tunnel: w492 -> [w506 _]
        tunnel: w489 -> [w505 _]
        tunnel: w487 -> [w504 _]
        tunnel: w486 -> [w503 _]
        frame False {
          n236 = case shown="\"Delete\"" w510 {
            tunnel: w506 -> [w514 w525]
            tunnel: w509 -> [_ w524]
            tunnel: w508 -> [w517 _]
            tunnel: w507 -> [w515 _]
            tunnel: w505 -> [w512 _]
            tunnel: w504 -> [_ w522]
            tunnel: w503 -> [_ w520]
            frame Default {
              n237 = case shown="Default" w515 {
                tunnel: ["OverwriteRelpace" ("sOption") "OverwriteInsert" ("sOption")] -> w516
                frame Default {
                }
                frame "Insert" {
                }
              }
              n238 = Build Array(w512) -> (w511:string[])
              n239 = Build Array(w517) -> (w513:T2[])
              n240 = call "CRYInsert Data to Listbox.vi"("OrgNames"=w511, "Type"=w514, "sOption"=w516, "Results"=w513) -> ()  [unwired: 7 in, 1 out]
            }
            frame "Delete" {
              n241 = flat-sequence {
                tunnel: w525 -> [w529]
                tunnel: w524 -> [w528]
                tunnel: [w527] -> w523
                tunnel: w522 -> [w527]
                tunnel: [w526] -> w521
                tunnel: w520 -> [w526]
                tunnel: w523 -> [w531]
                tunnel: w521 -> [w530]
                frame #0 {
                  n242 = call "CRYDelete Tree Items.vi"("Array"=w528, "Type"=w529) -> ()  [unwired: 2 in, 8 out]
                }
                frame #1 {
                  n243 = call "CRYGroup Manipulate Sub.vi"("sAction"="MakeGroupName", "sOption"="ChangeNum", "sData"=w531, "Tree in"=w530) -> ("Tree Out"=w535:refnum<vi>, "sData Out"=w536:string[])  [unwired: 3 in, 3 out]
                  n244 = call "CRYGroup Manipulate Sub.vi"("sAction"="DeleteEmptyGroup", "sData"=w536, "Tree in"=w535) -> ()  [unwired: 4 in, 5 out]
                }
              }
            }
          }
        }
        frame True {
        }
      }
    }
    frame "WFM" {
      n245 = case shown="Default" w682 {
        selector: w682 -> [w815 w821]
        tunnel: w674 -> [_ w820]
        tunnel: [_ w827] -> w684
        tunnel: w683 -> [_ w818]
        tunnel: w675 -> [_ w822]
        tunnel: [w815 w821] -> w681
        tunnel: [_ w817] -> w671
        frame "Delete" {
        }
        frame Default {
          n246 = call "CRYGet Curve Library Arr.vi"("Index"=w818, "sOption"="Some", "Type In"=w822) -> ("Waveforms"=w819:T4)  [unwired: 6 in, 2 out]
          n247 = Index Array(array=w819) -> (element=w825:T1)  [unwired: 1 in]
          n248 = Unbundle By Name(w825) -> ("Plot Settings"=w824:T7)
          n249 = global read "CRYCurve Library Global.vi" "StepOK"() -> (w816:bool)
          n250 = case shown="\"Replace_KeepName\", \"Replace_KeepStepNo\"" w821 {
            tunnel: w824 -> [w841 _]
            tunnel: w822 -> [_ w864]
            tunnel: [w840 w863] -> w823
            tunnel: w820 -> [w838 w862]
            tunnel: w816 -> [w837 _]
            frame "Replace_KeepName", "Replace_KeepStepNo" {
              n251 = case shown="True" w837 {
                tunnel: w838 -> [w842 w844]
                tunnel: [w842 w843] -> w839
                frame False {
                }
                frame True {
                  n252 = global read "CRYCurves Array Global.vi" "InsertWaveforms_Bk"() -> (w846:T4)
                  n253 = Unbundle By Name(w844) -> ("Name"=w845:string)
                  n254 = for {
                    tunnel: w846 -> [w854] mode=indexing
                    tunnel: [w853] -> w848 mode=indexing
                    n255 = Unbundle By Name(w854) -> ("Name"=w853:string)
                  }
                  n256 = Search 1D Array(1D array=w848, element=w845) -> (index of element=w847:i32)  [unwired: 1 in]
                  n257 = case shown="-1" w847 {
                    selector: w847 -> [w850 _]
                    tunnel: w846 -> [w851 _]
                    tunnel: [w849 w852] -> w843
                    tunnel: w844 -> [_ w852]
                    frame Default {
                      n258 = Index Array(array=w851, index=w850) -> (element=w849:T1)
                    }
                    frame -1 {
                    }
                  }
                }
              }
              n259 = Bundle By Name(cluster=w839, "Plot Settings"=w841) -> (w840:T1)
            }
            frame Default {
              n260 = call "CRYGet Next Color.vi"("Type"=w864) -> ("Color"=w858:u32)  [unwired: 10 out]
              n261 = Bundle By Name(cluster=w862, "Plot Settings.Color"=w858, "Plot Settings.Interpolation"=u8 2, "Plot Settings.Point Style"=u8 0, "Plot Settings.Line Style"=u8 0, "Plot Settings.Point Color"=w858, "Plot Settings.Line Width"=u8 0, "Plot Settings.Bar Plot Style"=u8 0, "Plot Settings.Fill To"=i16 -1) -> (w863:T1)
            }
          }
          n262 = case shown="Default" w821 {
            selector: w821 -> [w830 _]
            tunnel: [w833 w836] -> w827
            tunnel: w823 -> [w832 w836]
            tunnel: w818 -> [w829 _]
            tunnel: w822 -> [w831 _]
            tunnel: [w828 w835] -> w817
            frame "Insert" {
              n263 = Unbundle By Name(w832) -> ("Name"=w828:string)
              n264 = call "CRYMake Name.vi"("Type"=w831, "nData"=w829, "sAction"=w830, "Name In"=w828) -> ("Name Out"=w834:string)  [unwired: 6 in, 1 out]
              n265 = Bundle By Name(cluster=w832, "Name"=w834) -> (w833:T1)
            }
            frame Default {
              n266 = Unbundle By Name(w836) -> ("Name"=w835:string)
            }
          }
        }
      }
      n267 = flat-sequence {
        tunnel: w684 -> [w728]
        tunnel: w683 -> [w723]
        tunnel: w681 -> [w725]
        tunnel: [w725] -> w680
        tunnel: [w729] -> w679
        tunnel: [w727] -> w678
        tunnel: [w726] -> w676
        tunnel: [w730] -> w677
        tunnel: w668 -> [w722]
        tunnel: [w721] -> w672
        tunnel: w670 -> [w720]
        tunnel: [w719] -> w669
        frame #0 {
          n268 = case shown="\"Delete\"" w725 {
            tunnel: w728 -> [w736 _ w783 w798]
            tunnel: w723 -> [w743 w755 w771 w786]
            tunnel: [w732 w755 w771 w786] -> w729
            tunnel: [w736 _ w778 w791] -> w727
            tunnel: [w741 w756 w781 w796] -> w726
            tunnel: ["Insert" ("sOption") _ _ _] -> w730
            tunnel: enum16{"Curves", "Values", "Results", "WFM"}."WFM" ("Type") -> [w733 w757 w773 w788]
            tunnel: w722 -> [_ w750 _ _]
            tunnel: [_ w749 _ _] -> w721
            tunnel: w720 -> [_ _ _ w784]
            tunnel: [_ w748 _ _] -> w719
            frame "Insert", Default {
              n269 = Index Array(array=w743) -> (element=w742:i32)  [unwired: 1 in]
              n270 = call "CRYGlobal Manipulate.vi"("Type"=w733, "sAction"="GetSize") -> ("Type out"=w735:enum16{"Curves", "Values", "Results", "WFM"}, "nData out"=w740:i32[])  [unwired: 7 in, 5 out]
              n271 = Index Array(array=w740) -> (element=w738:i32)  [unwired: 1 in]
              n272 = Less Than 0?(x=w742) -> (x < 0?=w747:bool)
              n273 = Select(t=w738, s=w747, f=w742) -> (s? t:f=w744:i32)
              n274 = Unbundle By Name(w736) -> ("Name"=w746:string)
              n275 = Build Array(w744) -> (w732:i32[])
              n276 = Build Array(w736) -> (w734:T1[])
              n277 = Build Array(w746) -> (w741:string[])
              n278 = call "CRYGlobal Manipulate.vi"("Type"=w735, "sOption"="byIndex", "sAction"="Insert", "WFM"=w734, "nData"=w732) -> ()  [unwired: 4 in, 7 out]
            }
            frame "Delete" {
              n279 = flat-sequence {
                tunnel: w757 -> [w760]
                tunnel: w750 -> [w762]
                tunnel: w755 -> [w761]
                tunnel: [w760] -> w758
                tunnel: [w759] -> w749
                tunnel: [w766] -> w756
                tunnel: w758 -> [w765]
                tunnel: w755 -> [w764]
                frame #0 {
                  n280 = call "CRYTree Manuplate.vi"("Type"=w760, "sAction"="GetViewNumbyGlobalNum", "nData"=w761, "Tree in"=w762) -> ("nData Out"=w759:i32[])  [unwired: 4 in, 3 out]
                }
                frame #1 {
                  n281 = call "CRYGlobal Manipulate.vi"("Type"=w765, "sOption"="byIndex", "sAction"="Delete", "nData"=w764) -> ("sData Out"=w766:string[])  [unwired: 5 in, 6 out]
                }
              }
              n282 = call "CRYTree Manuplate.vi"("sAction"="GetItemNames", "nData"=w749, "Tree in"=w750) -> ("sData Out"=w751:string[], "Tree Out"=w752:refnum<vi>)  [unwired: 5 in, 2 out]
              n283 = call "CRYTree Manuplate.vi"("sData"=w751, "sAction"="GetAllParents", "Tree in"=w752) -> ("sData Out"=w748:string[])  [unwired: 5 in, 3 out]
            }
            frame "Replace_KeepName" {
              n284 = call "CRYGlobal Manipulate.vi"("Type"=w773, "sOption"="byIndex", "sAction"="GetGlobal", "nData"=w771) -> ("Type out"=w777:enum16{"Curves", "Values", "Results", "WFM"}, "WFM Out"=w774:T1[])  [unwired: 5 in, 5 out]
              n285 = Index Array(array=w774) -> (element=w776:T1)  [unwired: 1 in]
              n286 = Unbundle By Name(w776) -> ("Name"=w782:string, "AutoProtect"=w769:bool)
              n287 = Bundle By Name(cluster=w783, "Name"=w782, "AutoProtect"=w769) -> (w778:T1)
              n288 = Build Array(w778) -> (w775:T1[])
              n289 = call "CRYGlobal Manipulate.vi"("Type"=w777, "sOption"="byIndex", "sAction"="Replace", "WFM"=w775, "nData"=w771) -> ()  [unwired: 4 in, 7 out]
              n290 = Build Array(w782) -> (w781:string[])
            }
            frame "Replace_KeepStepNo" {
              n291 = call "CRYGlobal Manipulate.vi"("Type"=w788, "sOption"="byIndex", "sAction"="GetGlobal", "nData"=w786) -> ("Type out"=w793:enum16{"Curves", "Values", "Results", "WFM"}, "WFM Out"=w792:T1[])  [unwired: 5 in, 5 out]
              n292 = Index Array(array=w792) -> (element=w789:T1)  [unwired: 1 in]
              n293 = case shown="False" w784 {
                tunnel: w798 -> [w803 w814]
                tunnel: [w800 w813] -> w797
                tunnel: [w804 w812] -> w791
                tunnel: w789 -> [w802 w811]
                frame True {
                  n294 = Unbundle By Name(w802) -> ("Name"=w799:string)
                  n295 = Unbundle By Name(w803) -> ("Name"=w801:string)
                  n296 = flat-sequence {
                    tunnel: [w808] -> w804
                    tunnel: w802 -> [w807]
                    tunnel: w801 -> [w806]
                    tunnel: [w805] -> w800
                    tunnel: w799 -> [w805]
                    frame #0 {
                      n297 = Bundle By Name(cluster=w807, "Name"=w806) -> (w808:T1)
                    }
                  }
                }
                frame False {
                  n298 = Unbundle By Name(w811) -> ("Step No."=w809:i32, "Name"=w813:string, "AutoProtect"=w810:bool)
                  n299 = Bundle By Name(cluster=w814, "Step No."=w809, "Name"=w813, "AutoProtect"=w810) -> (w812:T1)
                }
              }
              n300 = Build Array(w791) -> (w790:T1[])
              n301 = call "CRYGlobal Manipulate.vi"("Type"=w793, "sOption"="byIndex", "sAction"="Replace", "WFM"=w790, "nData"=w786) -> ()  [unwired: 4 in, 7 out]
              n302 = Build Array(w797) -> (w796:string[])
            }
          }
        }
      }
      n303 = case shown="False" w673 {
        tunnel: w680 -> [w692 _]
        tunnel: w672 -> [w691 _]
        tunnel: w678 -> [w690 _]
        tunnel: w677 -> [w689 _]
        tunnel: w675 -> [w688 _]
        tunnel: w671 -> [w687 _]
        tunnel: w669 -> [w686 _]
        tunnel: w668 -> [w685 _]
        frame False {
          n304 = case shown="\"Delete\"" w692 {
            tunnel: w688 -> [w696 w707]
            tunnel: w691 -> [_ w706]
            tunnel: w690 -> [w699 _]
            tunnel: w689 -> [w697 _]
            tunnel: w687 -> [w694 _]
            tunnel: w686 -> [_ w704]
            tunnel: w685 -> [_ w702]
            frame Default {
              n305 = case shown="\"Insert\"" w697 {
                tunnel: ["OverwriteRelpace" ("sOption") "OverwriteInsert" ("sOption")] -> w698
                frame Default {
                }
                frame "Insert" {
                }
              }
              n306 = Build Array(w699) -> (w695:T1[])
              n307 = Build Array(w694) -> (w693:string[])
              n308 = call "CRYInsert Data to Listbox.vi"("OrgNames"=w693, "Type"=w696, "sOption"=w698, "Waveforms"=w695) -> ()  [unwired: 7 in, 1 out]
            }
            frame "Delete" {
              n309 = flat-sequence {
                tunnel: w707 -> [w711]
                tunnel: w706 -> [w710]
                tunnel: [w709] -> w705
                tunnel: w704 -> [w709]
                tunnel: [w708] -> w703
                tunnel: w702 -> [w708]
                tunnel: w705 -> [w713]
                tunnel: w703 -> [w712]
                frame #0 {
                  n310 = call "CRYDelete Tree Items.vi"("Array"=w710, "Type"=w711) -> ()  [unwired: 2 in, 8 out]
                }
                frame #1 {
                  n311 = call "CRYGroup Manipulate Sub.vi"("sAction"="MakeGroupName", "sOption"="ChangeNum", "sData"=w713, "Tree in"=w712) -> ("Tree Out"=w717:refnum<vi>, "sData Out"=w718:string[])  [unwired: 3 in, 3 out]
                  n312 = call "CRYGroup Manipulate Sub.vi"("sAction"="DeleteEmptyGroup", "sData"=w718, "Tree in"=w717) -> ()  [unwired: 4 in, 5 out]
                }
              }
            }
          }
        }
        frame True {
        }
      }
    }
  }
  "Inserted index" <- w23
  "Name Out" <- w21
